vi "791flourescence.vi"() -> ()   [LabVIEW 2009]
uses:
  <vilib>/Utility/error.llb/DialogType.ctl
  <vilib>/DAQmx/configure/timing.llb/DAQmx Timing (Sample Clock).vi
  <vilib>/DAQmx/create/channels.llb/DAQmx Create Channel (CI-Count Edges).vi
  <vilib>/DAQmx/write.llb/DAQmx Write (Digital Wfm 1Chan NSamp).vi
  <vilib>/DAQmx/configure/timing.llb/DAQmx Timing (Implicit).vi
  <vilib>/DAQmx/create/channels.llb/DAQmx Create Channel (CO-Pulse Generation-Frequency).vi
  <vilib>/DAQmx/create/channels.llb/DAQmx Create Channel (DO-Digital Output).vi
  <vilib>/Waveform/DWDTOps.llb/DWDT Digital Size.vi
  <vilib>/DAQmx/read.llb/DAQmx Read (Counter 1D U32 1Chan NSamp).vi
  Program Files/National Instruments/LabVIEW 2009/resource/objmgr/daqmx.rc
panel:
  out "Waveform Graph":u32[](graph)
  in  "Runs":i32=100000
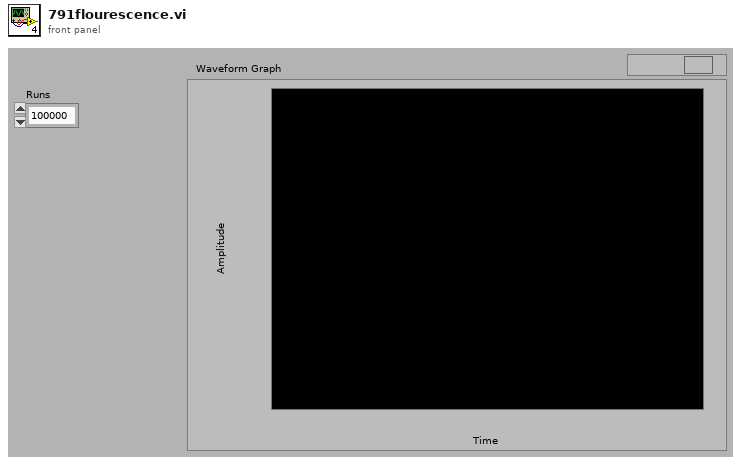
[diagram p1: front panel]
types:
  T1 = enum16{"open", "replace", "create", "open or create", "replace or create", "replace or create with confirmation"}
  T2 = typedef "DialogType.ctl" = u16
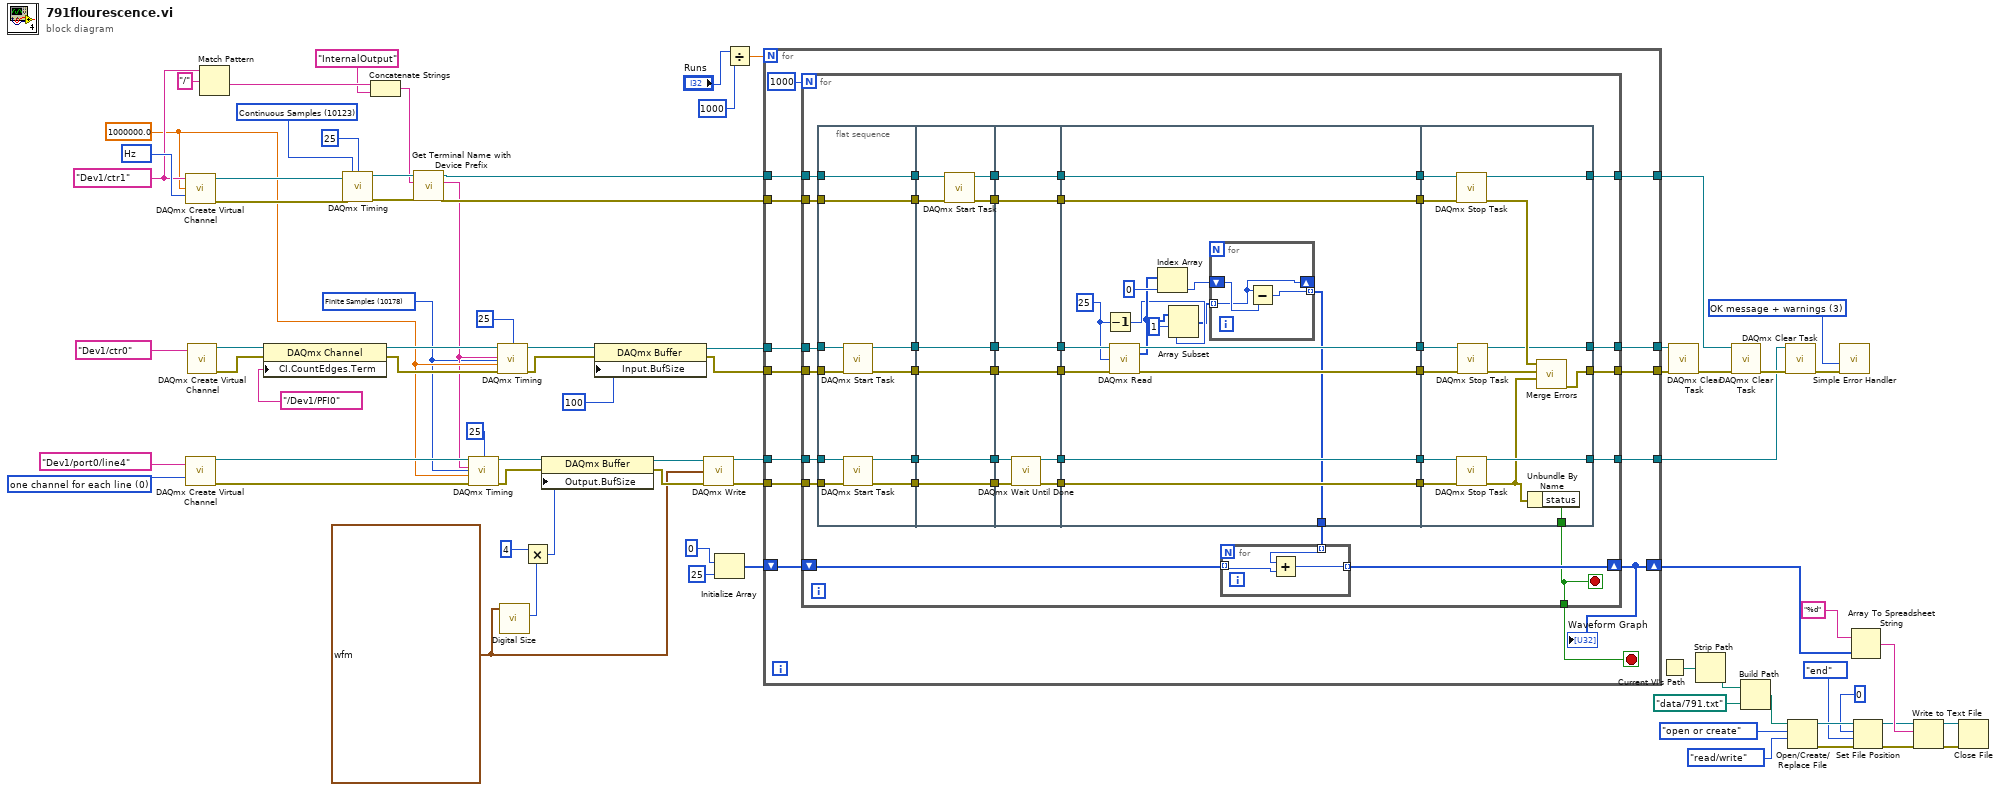
[diagram p0: block diagram]
diagram:
  w26 = 10178 items=["Finite Samples"=10178, "Continuous Samples"=10123, "Hardware Timed Single Point"=12522] ("sample mode")
  w36 = digitalwaveform {"t0"=timestamp(0 s since 1904-01-01), "dt"=1e-06, "Y"={"transitions"=[], "data"=[[1], [1], [1], [1], [0], [0], [0], [0], [1], [1], [1], [1], [0], [0], [0], [0], [1], [1], [1], [1], [0], [0], [0], [0], [0]]}, "error"={"status"=FALSE, "code"=37421928, "source"=""}} ("data")
  w46 = T2 3 items=["no dialog", "OK message", "continue or stop message", "OK message + warnings", "continue/stop + warnings"] ("type of dialog (OK msg:1)")
  w50 = 1000000.0 ("frequency")
  w57 = 0 items=["one channel for each line", "one channel for all lines"] ("line grouping")
  w60 = tag "Dev1/ctr1" ("counter")
  w61 = 10373 items=["Hz"=10373] ("units")
  w55 = 10123 items=["Finite Samples"=10178, "Continuous Samples"=10123] ("sample mode")
  n1 = call-poly <vilib>:"DAQmx Create Virtual Channel.vi"("frequency"=w50, "counter"=w60, "units"=w61) -> ("task out"=w68:refnum<k21>, "error out"=w67:errorcluster)  [unwired: 11 in]
  n2 = call-poly <vilib>:"DAQmx Create Virtual Channel.vi"("lines"=tag "Dev1/port0/line4", "line grouping"=w57) -> ("task out"=w59:refnum<k21>, "error out"=w58:errorcluster)  [unwired: 12 in]
  n3 = call-poly <vilib>:"DAQmx Create Virtual Channel.vi"("counter"=tag "Dev1/ctr0") -> ("task out"=w72:refnum<k21>, "error out"=w71:errorcluster)  [unwired: 13 in]
  n4 = Match Pattern(string=w60, regular expression="/") -> (after substring=w64:string)  [unwired: 1 in, 3 out]
  n5 = property class="DAQmx Channel"(reference=w72, error in=w71, "CI.CountEdges.Term"=tag "/Dev1/PFI0") -> (reference out=w74:refnum<k21>, error out=w73:errorcluster)
  n6 = call-poly <vilib>:"DAQmx Timing.vi"("task/channels in"=w68, "sample mode"=w55, "samples per channel"=25, "error in"=w67) -> ("task out"=w66:refnum<k21>, "error out"=w69:errorcluster)  [unwired: 10 in]
  n7 = Concatenate Strings(w64, "InternalOutput" ("Local Terminal Name")) -> (w62:string)
  n8 = call "Get Terminal Name with Device Prefix.vi"("error in (no error)"=w69, "Local Terminal Name"=w62, "task/channels in"=w66) -> ("error out"=w51:errorcluster, "Terminal Name with Device Prefix"=w41:tag, "task out"=w52:refnum<k21>)  [unwired: 6 in]
  n9 = call-poly <vilib>:"DAQmx Timing.vi"("task/channels in"=w59, "sample mode"=w26, "samples per channel"=25, "rate"=w50, "source"=w41, "error in"=w58) -> ("task out"=w40:refnum<k21>, "error out"=w39:errorcluster)  [unwired: 8 in]
  n10 = call-poly <vilib>:"DAQmx Timing.vi"("task/channels in"=w74, "sample mode"=w26, "samples per channel"=25, "rate"=w50, "source"=w41, "error in"=w73) -> ("task out"=w32:refnum<k21>, "error out"=w31:errorcluster)  [unwired: 8 in]
  n11 = call-poly <vilib>:"Digital Size.vi"("digital waveform in"=w36) -> ("number of samples"=w35:i32)  [unwired: 7 in, 3 out]
  n12 = Multiply(x=4, y=w35) -> (x*y=w33:i32)
  n13 = property class="DAQmx Buffer"(reference=w40, error in=w39, "Output.BufSize"=w33) -> (reference out=w37:refnum<k21>, error out=w38:errorcluster)
  n14 = property class="DAQmx Buffer"(reference=w32, error in=w31, "Input.BufSize"=u32 100 ("Output.BufSize")) -> (reference out=w30:refnum<k21>, error out=w29:errorcluster)
  n15 = call-poly <vilib>:"DAQmx Write.vi"("task/channels in"=w37, "data"=w36, "error in"=w38) -> ("task out"=w54:refnum<k21>, "error out"=w53:errorcluster)  [unwired: 10 in, 1 out]
  n16 = Initialize Array(0, 25 ("dimension size")) -> (w22:i32[])
  n17 = Divide(x="Runs", y=1000) -> (x/y=w1:dbl)
  n18 = for {
    N: w1 -> [_]
    tunnel: w54 -> [w89]
    tunnel: w53 -> [w88]
    tunnel: w52 -> [w87]
    tunnel: w51 -> [w86]
    tunnel: [w85] -> w45
    tunnel: [w84] -> w44
    tunnel: [w83] -> w43
    tunnel: [w82] -> w42
    tunnel: w30 -> [w81]
    tunnel: w29 -> [w80]
    shift-right: [w76] -> w17
    shift-left: w22 -> [w79]
    stop <- w77 stop-if-true
    n19 = for {
      N: 1000 -> [_]
      tunnel: w89 -> [w103]
      tunnel: w88 -> [w102]
      tunnel: w87 -> [w101]
      tunnel: w86 -> [w100]
      tunnel: [w99] -> w85
      tunnel: [w98] -> w84
      tunnel: [w97] -> w83
      tunnel: [w96] -> w82
      tunnel: w81 -> [w95]
      tunnel: w80 -> [w94]
      tunnel: [w90] -> w77
      shift-right: [w91] -> w76
      shift-left: w79 -> [w93]
      stop <- w90 stop-if-true
      n20 = flat-sequence {
        tunnel: w95 -> [w140]
        tunnel: w94 -> [w139]
        tunnel: w103 -> [w138]
        tunnel: w102 -> [w137]
        tunnel: [w136] -> w127
        tunnel: w101 -> [w136]
        tunnel: [w135] -> w126
        tunnel: w100 -> [w135]
        tunnel: [w134] -> w125
        tunnel: [w133] -> w124
        tunnel: [w132] -> w123
        tunnel: [w131] -> w122
        tunnel: w127 -> [w148]
        tunnel: w126 -> [w147]
        tunnel: [w146] -> w121
        tunnel: w125 -> [w146]
        tunnel: [w145] -> w120
        tunnel: w124 -> [w145]
        tunnel: [w144] -> w119
        tunnel: w123 -> [w144]
        tunnel: [w143] -> w118
        tunnel: w122 -> [w143]
        tunnel: [w142] -> w117
        tunnel: [w141] -> w116
        tunnel: [w156] -> w115
        tunnel: w121 -> [w156]
        tunnel: [w155] -> w114
        tunnel: w120 -> [w155]
        tunnel: w119 -> [w154]
        tunnel: w118 -> [w153]
        tunnel: [w152] -> w113
        tunnel: [w151] -> w112
        tunnel: [w150] -> w111
        tunnel: w117 -> [w150]
        tunnel: [w149] -> w110
        tunnel: w116 -> [w149]
        tunnel: w115 -> [w172]
        tunnel: w114 -> [w171]
        tunnel: [w170] -> w109
        tunnel: [w169] -> w108
        tunnel: [w168] -> w107
        tunnel: w113 -> [w168]
        tunnel: [w167] -> w106
        tunnel: w112 -> [w167]
        tunnel: [w166] -> w105
        tunnel: w111 -> [w166]
        tunnel: [w165] -> w104
        tunnel: w110 -> [w165]
        tunnel: [w157] -> w92
        tunnel: w109 -> [w189]
        tunnel: w108 -> [w188]
        tunnel: w107 -> [w187]
        tunnel: w106 -> [w186]
        tunnel: w105 -> [w185]
        tunnel: w104 -> [w184]
        tunnel: [w181] -> w99
        tunnel: [w180] -> w98
        tunnel: [w179] -> w97
        tunnel: [w178] -> w96
        tunnel: [w176] -> w90
        frame #0 {
          n21 = call <vilib>:"DAQmx Start Task.vi"("task/channels in"=w140, "error in"=w139) -> ("task out"=w134:refnum<k21>, "error out"=w133:errorcluster)  [unwired: 12 in]
          n22 = call <vilib>:"DAQmx Start Task.vi"("task/channels in"=w138, "error in"=w137) -> ("task out"=w132:refnum<k21>, "error out"=w131:errorcluster)  [unwired: 12 in]
        }
        frame #1 {
          n23 = call <vilib>:"DAQmx Start Task.vi"("task/channels in"=w148, "error in"=w147) -> ("task out"=w142:refnum<k21>, "error out"=w141:errorcluster)  [unwired: 12 in]
        }
        frame #2 {
          n24 = call <vilib>:"DAQmx Wait Until Done.vi"("task/channels in"=w154, "error in"=w153) -> ("task out"=w151:refnum<k21>, "error out"=w152:errorcluster)  [unwired: 12 in]
        }
        frame #3 {
          w160 = 25 ("number of samples per channel")
          n25 = Decrement(x=w160) -> (x-1=w159:i32)
          n26 = call-poly <vilib>:"DAQmx Read.vi"("task/channels in"=w172, "number of samples per channel"=w160, "error in"=w171) -> ("task out"=w169:refnum<k21>, "data"=w162:u32[], "error out"=w170:errorcluster)  [unwired: 10 in]
          n27 = Index Array(array=w162, index=0) -> (element=w163:u32)
          n28 = Array Subset(array=w162, index=1, length=w159) -> (w158:u32[])
          n29 = for {
            tunnel: [w175] -> w157 mode=indexing
            shift-right: [w173] -> _
            shift-left: w163 -> [w174]
            tunnel: w158 -> [w173] mode=indexing
            n30 = Subtract(x=w173, y=w174) -> (x-y=w175:u32)
          }
        }
        frame #4 {
          n31 = call <vilib>:"DAQmx Stop Task.vi"("task/channels in"=w185, "error in"=w184) -> ("task out"=w179:refnum<k21>, "error out"=w183:errorcluster)  [unwired: 12 in]
          n32 = call <vilib>:"DAQmx Stop Task.vi"("task/channels in"=w186, "error in"=w187) -> ("task out"=w178:refnum<k21>, "error out"=w177:errorcluster)  [unwired: 12 in]
          n33 = call <vilib>:"DAQmx Stop Task.vi"("task/channels in"=w188, "error in"=w189) -> ("task out"=w180:refnum<k21>, "error out"=w182:errorcluster)  [unwired: 12 in]
          n34 = Unbundle By Name(w177) -> ("status"=w176:bool)
          n35 = call <vilib>:"Merge Errors.vi"("error in 3 (no error)"=w177, "error in 2 (no error)"=w182, "error in 1 (no error)"=w183) -> ("error out"=w181:errorcluster)  [unwired: 4 in]
        }
      }
      n36 = for {
        tunnel: w93 -> [w130] mode=indexing
        tunnel: w92 -> [w129] mode=indexing
        tunnel: [w128] -> w91 mode=indexing
        n37 = Add(x=w129, y=w130) -> (x+y=w128:u32)
      }
    }
    "Waveform Graph" <- w76
  }
  n38 = Current VI's Path() -> (path=w11:path)
  n39 = call <vilib>:"DAQmx Clear Task.vi"("task in"=w44, "error in"=w45) -> ("error out"=w49:errorcluster)  [unwired: 13 in]
  n40 = Strip Path(path=w11) -> (stripped path=w10:path)  [unwired: 1 out]
  n41 = call <vilib>:"DAQmx Clear Task.vi"("task in"=w43, "error in"=w49) -> ("error out"=w48:errorcluster)  [unwired: 13 in]
  n42 = Build Path(base path=w10, name or relative path=path "data/791.txt" ("file path (use dialog)")) -> (appended path=w12:path)
  n43 = call <vilib>:"DAQmx Clear Task.vi"("task in"=w42, "error in"=w48) -> ("error out"=w47:errorcluster)  [unwired: 13 in]
  n44 = Open/Create/Replace File(file path (use dialog)=w12, operation (0:open)=T1."open or create", access (0:read/write)=enum16{"read/write", "read-only", "write-only"}."read/write") -> (refnum out=w8:refnum<file>, error out=w9:errorcluster)  [unwired: 3 in, 1 out]
  n45 = call <vilib>:"Simple Error Handler.vi"("type of dialog (OK msg:1)"=w46, "error in (no error)"=w47) -> ()  [unwired: 3 in, 5 out]
  n46 = Array To Spreadsheet String(array=w17, 3:"%d" ("format string")) -> (spreadsheet string=w16:string)  [unwired: 1 in]
  n47 = Set File Position(offset (in bytes) (0)=i64 0, refnum=w8, from (0:start)=enum16{"start", "end", "current"}."end", error in=w9) -> (refnum out=w6:refnum<file>, error out=w7:errorcluster)
  n48 = Write to Text File(file (use dialog)=w6, text=w16, error in=w7) -> (refnum out=w15:refnum<file>, error out=w14:errorcluster)  [unwired: 1 in, 1 out]
  n49 = Close File(refnum=w15, error in=w14) -> ()  [unwired: 2 out]
